vi "SwissSPAD Live_Reorder SS3 Gate Image Data.vi"(6 "X Resolution (500)":i32=500, 8 "Error In":errorcluster, 11 "Interlaced Gate (512x250)":u8[][](array[numeric])) -> (0 "Error Out":errorcluster, 3 "De-interlaced Gate (500x250)":u8[][](array[numeric]))   [LabVIEW 2021]
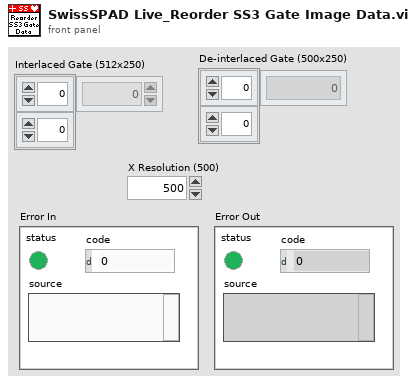
[diagram p1: front panel]
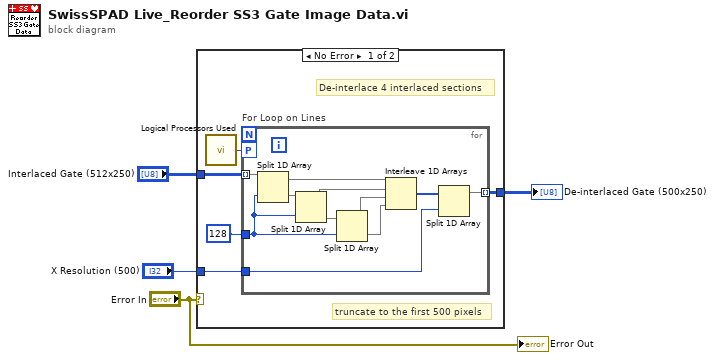
[diagram p0: block diagram]
diagram:
  n1 = case shown="No Error" "Error In" {
    tunnel: "X Resolution (500)" -> [w8 _]
    tunnel: [w7 w21] -> w3
    tunnel: "Interlaced Gate (512x250)" -> [w6 w21]
    frame No Error {
      # "truncate to the first 500 pixels"
      # "De-interlace 4 interlaced sections"
      n2 = call "Logical Processors Used.vi"() -> ("# Logical Processor Used"=w5:i32)  [unwired: 6 in]
      n3 = for "For Loop on Lines" {
        tunnel: w6 -> [w20] mode=indexing
        tunnel: 128 -> [w17]
        tunnel: [w10] -> w7 mode=indexing
        workers-P: w5 -> [_]
        tunnel: w8 -> [w11]
        n4 = Split 1D Array(array=w20, index=w17) -> (first subarray=w16:u8[], second subarray=w19:u8[])
        n5 = Split 1D Array(array=w19, index=w17) -> (first subarray=w15:u8[], second subarray=w18:u8[])
        n6 = Split 1D Array(array=w18, index=w17) -> (first subarray=w14:u8[], second subarray=w13:u8[])
        n7 = Interleave 1D Arrays(w16, w15, w14, w13) -> (w12:u8[])
        n8 = Split 1D Array(array=w12, index=w11) -> (first subarray=w10:u8[])  [unwired: 1 out]
      }
    }
    frame Error {
    }
  }
  "De-interlaced Gate (500x250)" <- w3
  "Error Out" <- "Error In"
